vi "Data types.vi"() -> ()   [LabVIEW 2014]
panel:
  out "Boolean 2":bool
  out "String 2":string
  out "Floating point 2":dbl
  out "Integer 2":dbl
  in  "String":string
  in  "Floating point":dbl
  in  "Boolean":bool
  in  "Integer":dbl
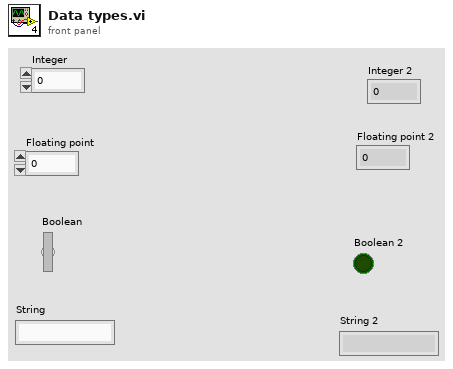
[diagram p1: front panel]
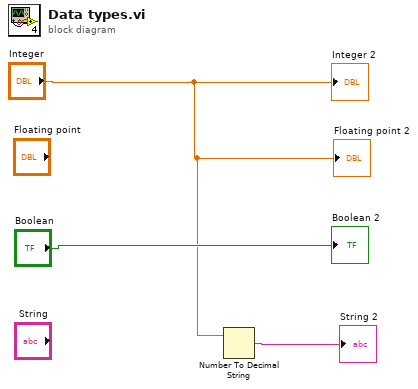
[diagram p0: block diagram]
diagram:
  n1 = Number To Decimal String(number="Integer") -> (decimal integer string=→"String 2":string)  [unwired: 1 in]
  "Integer 2" <- "Integer"
  "Floating point 2" <- "Integer"
  "Boolean 2" <- "Boolean"
